vi "hidSPD Open Multi Sessions.vi"(8 "error in (no error)":errorcluster, 11 "devices list":T3[](array[typedef])) -> (0 "error out":errorcluster, 3 "spdDevSessions out":T1[](array[typedef]) {"hidSPD.Controller"."HV_bias" format="%#_6p, V"; "hidSPD.Controller"."TSet" format="%#_6p, DegC"})   [LabVIEW 2018, in "hidSPDLibForLabView.lvlib"]
uses:
  hidSPDLibForLabView.lvlib
  hidSPD Controls/hidSPD HidDevInfo.ctl
  hidSPD Controls/hidSPD Device Session.ctl
  hidSPD Controls/hidSPD Controller.ctl
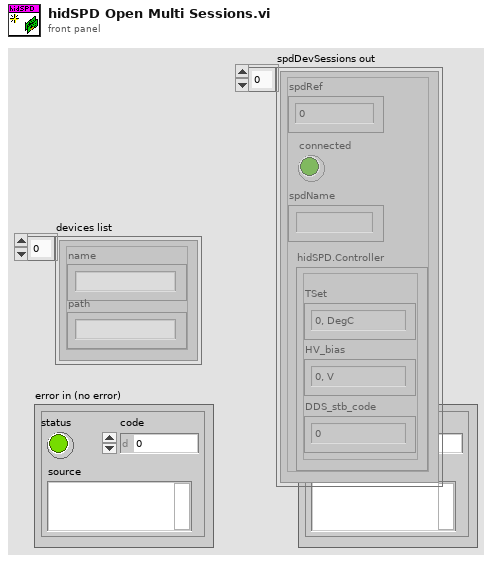
[diagram p1: front panel]
types:
  T1 = typedef "hidSPDLibForLabView.lvlib/hidSPD Device Session.ctl" = cluster{"spdRef":u64, "connected":bool, "spdName":string, "hidSPD.Controller":T2}
  T2 = typedef "hidSPDLibForLabView.lvlib/hidSPD Controller.ctl" = cluster{"TSet":sgl, "HV_bias":sgl, "DDS_stb_code":u16}
  T3 = typedef "hidSPDLibForLabView.lvlib/hidSPD HidDevInfo.ctl" = cluster{"name":string, "path":string}
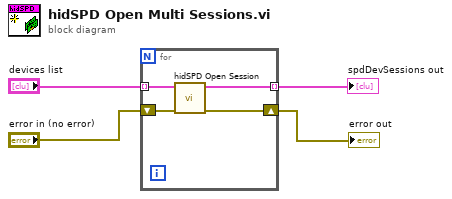
[diagram p0: block diagram]
diagram:
  n1 = for {
    tunnel: "devices list" -> [w8] mode=indexing
    shift-right: [w5] -> w2
    shift-left: "error in (no error)" -> [w7]
    tunnel: [w6] -> w1 mode=indexing
    n2 = call "hidSPD Open Session.vi"("error in (no error)"=w7, "HidDevInfo"=w8) -> ("error out"=w5:errorcluster, "spdDevSession out"=w6:T1)  [unwired: 8 in]
  }
  "error out" <- w2
  "spdDevSessions out" <- w1
